vi "PPMS Dashboard.glb.vi"() -> ()   [LabVIEW 2011]
panel:
  out "i X 2":cluster{"Y":dbl[], "Y":dbl[]}[](graph)
  in  "Tab Control":enum32{"I-V Curves", "Cooldown/Warmup"}(tab)
  out "Temp vs Time":cluster{"Y":dbl[], "Y":dbl[]}[](graph)
  out "Zx 3":cluster{"Y":dbl[], "Y":dbl[]}[](graph)
  out "Input signal":dbl[][](graph)
  out "Two terminal IV":cluster{dbl[], dbl[]}(graph)
  out "Temperature (K)":dbl=0.049957
  out "Field (Oe)":dbl=-0.164
  in  "Vsgw":dbl
  in  "Vsg2":dbl
  in  "Vsg1":dbl
  in  "Comments":string="SSA02610k.20121022\nScale parameters:\nVsg1: 120mV/-50mV\nVsg2: 160mV/-35mV\nVsgw: 40mV/-20mV\nVbg=0 V\nfield=0\nmounted Vertically\n\nVsg2, Vsg1, Vsgw sweep separately -2.5 to +2 in .22 step\n3mV amplitude +400uVDC, sawtooth, 5s, 1 curve per gate\nscan priority (fast to slow) Vsg2>Vsg1>Vsgw\n"
  out "I vs V":cluster{dbl[], dbl[]}[](graph)
  out "Last Scan Image":T1(plugin-control)
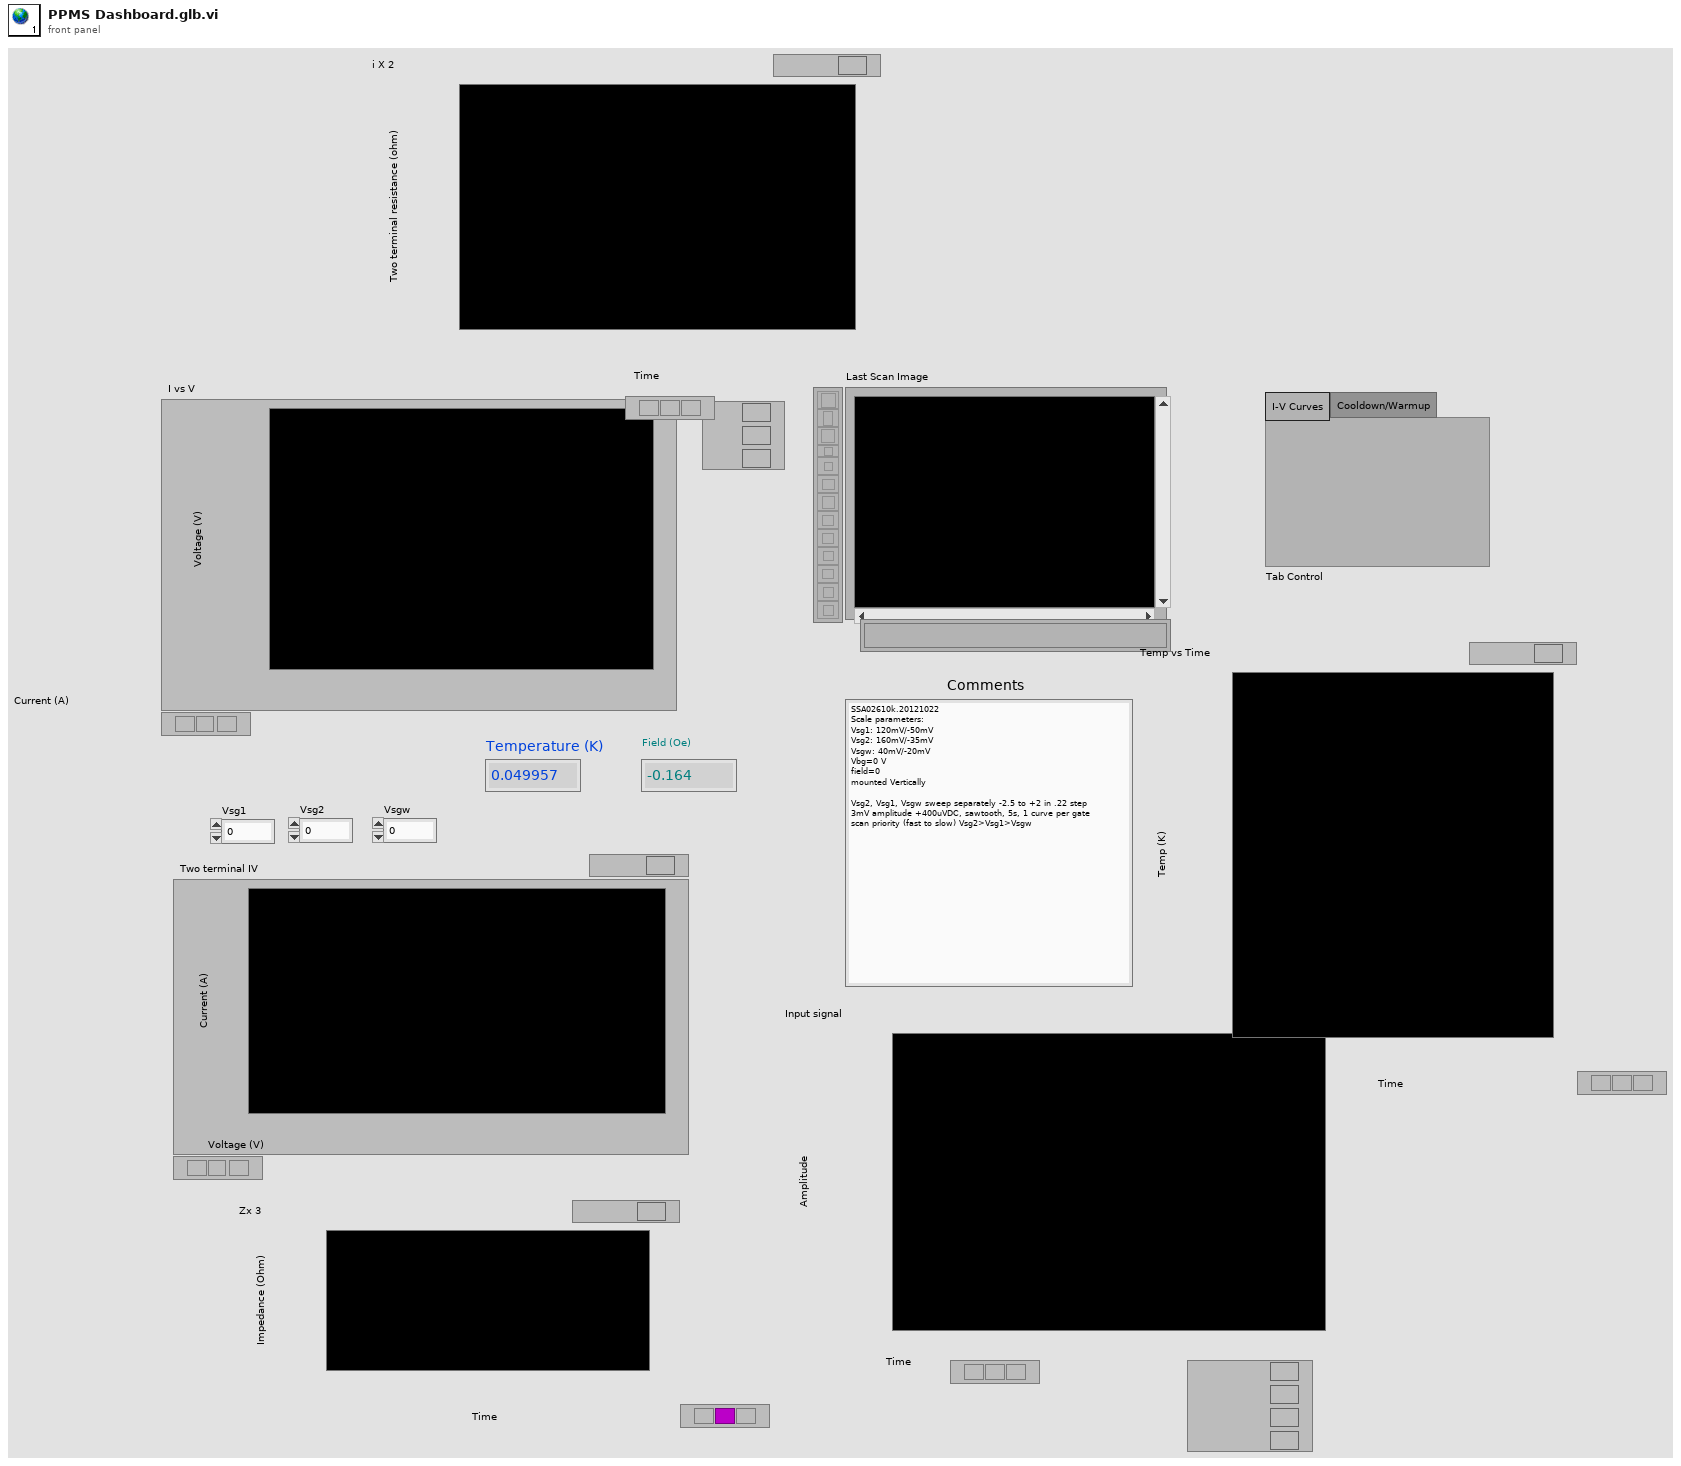
[diagram p1: front panel]
types:
  T1 = typedef "IMAQ Image.ctl" = refnum<image>
diagram:
